vi "deployScriptLinuxDesktop.vi"() -> ()   [LabVIEW 2016]
uses:
  Typedefs/Linux Desktop.ctl
  Typedefs/cRIO.ctl
  FileTransfer/FileTransfer.lvclass
  Typedefs/Item For Copy Selection.ctl
  FileTransfer/FileTransfer.lvclass/FileTransfer.ctl
panel:
  out "error out":errorcluster
  in  "error in (no error)":errorcluster
  in  "cRIO":T1={"Username"="admin", "IP Address"="140.252.33.38", "Path to ts_opensplice target"=path "/usr", "Path to ts_sal target"=path "/usr"}
  in  "Linux Desktop":T2={"Username"="plotz", "IP Address"="127.0.0.1", "Path to ts_opensplice source"=path "/home/plotz/lsst_ts/ts_opensplice", "Path to ts_sal source"=path "/home/plotz/lsst_ts/ts_sal"}
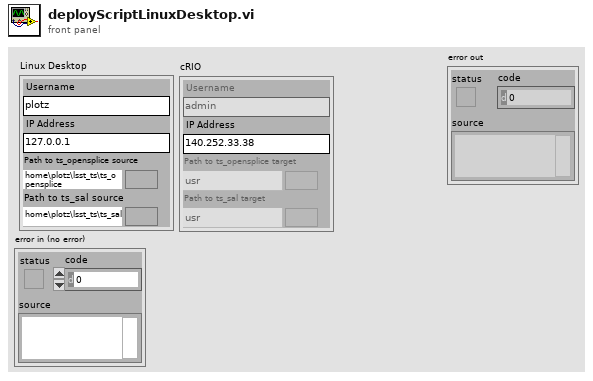
[diagram p1: front panel]
types:
  T1 = typedef "cRIO.ctl" = cluster{"Username":string, "IP Address":string, "Path to ts_opensplice target":path, "Path to ts_sal target":path}
  T2 = typedef "Linux Desktop.ctl" = cluster{"Username":string, "IP Address":string, "Path to ts_opensplice source":path, "Path to ts_sal source":path}
  T3 = typedef "Item For Copy Selection.ctl" = enum16{"ts_opensplice", "ts_sal"}
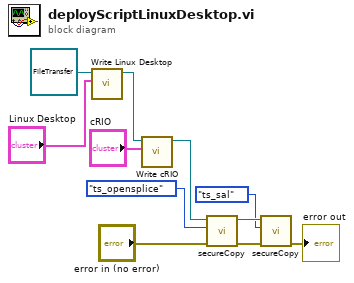
[diagram p0: block diagram]
diagram:
  n1 = call "Write Linux Desktop.vi"("Linux Desktop"="Linux Desktop", "FileTransfer in"=refnum<class "FileTransfer.lvclass"> refnum) -> ("FileTransfer out"=w10:refnum<class "FileTransfer.lvclass">)  [unwired: 9 in]
  n2 = call "Write cRIO.vi"("cRIO"="cRIO", "FileTransfer in"=w10) -> ("FileTransfer out"=w7:refnum<class "FileTransfer.lvclass">)  [unwired: 9 in]
  n3 = call "secureCopy.vi"("error in (no error)"="error in (no error)", "Item For Copy Selection"=Item_For_Copy_Selection."ts_opensplice", "FileTransfer in"=w7) -> ("error out"=w2:errorcluster, "FileTransfer out"=w5:refnum<class "FileTransfer.lvclass">)  [unwired: 7 in]
  n4 = call "secureCopy.vi"("error in (no error)"=w2, "Item For Copy Selection"=Item_For_Copy_Selection."ts_sal", "FileTransfer in"=w5) -> ("error out"=→"error out":errorcluster)  [unwired: 7 in, 1 out]
